vi "NIIE_Origin_or_TempCoordinate.vi"(9 "Temp Coord":T1, 11 "Origin":T1) -> (3 "Origin Out":T1, 7 "Temp? Out":bool)   [LabVIEW 2021]
uses:
  <vilib>/Utility/miscctls.llb/LVPoint32TypeDef.ctl
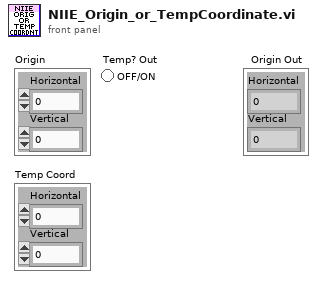
[diagram p1: front panel]
types:
  T1 = typedef "LVPoint32TypeDef.ctl" = cluster{"Horizontal":i32, "Vertical":i32}
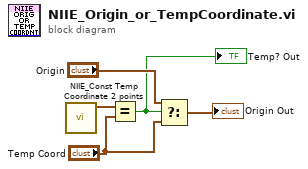
[diagram p0: block diagram]
diagram:
  n1 = call "NIIE_Const Temp Coordinate 2 points.vi"() -> ("Const Temp Coordinate"=w5:T1)  [unwired: 11 out]
  n2 = Equal?(x=w5, y="Temp Coord") -> (x = y?=w1:bool)
  "Temp? Out" <- w1
  n3 = Select(t="Origin", s=w1, f="Temp Coord") -> (s? t:f=→"Origin Out":T1)
